vi "OpenProject.vi"() -> ()   [LabVIEW 2020]
uses:
  <vilib>/Wiresmith Technology/G CLI/CLI Class/CLI.lvclass
panel:
  out "String":string
  out "Error out":errorcluster
  in  "Project_Path":path=path "C:/Workspace/Git/PVS_2.0/SourceCode/PVS_BE/Projects/PVS_BE.lvproj"
  in  "Error_In":errorcluster
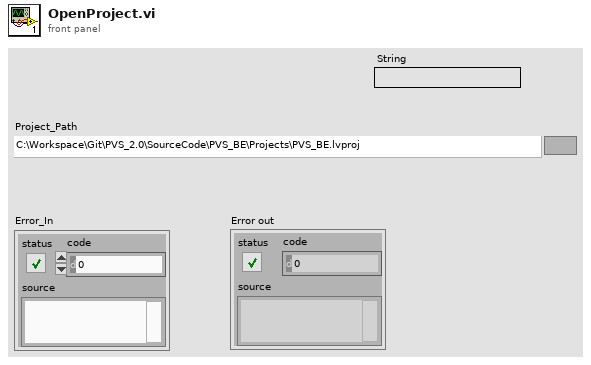
[diagram p1: front panel]
types:
  T1 = enum32{"Invalid", "Standard", "Closed", "Hidden", "Minimized", "Maximized"}
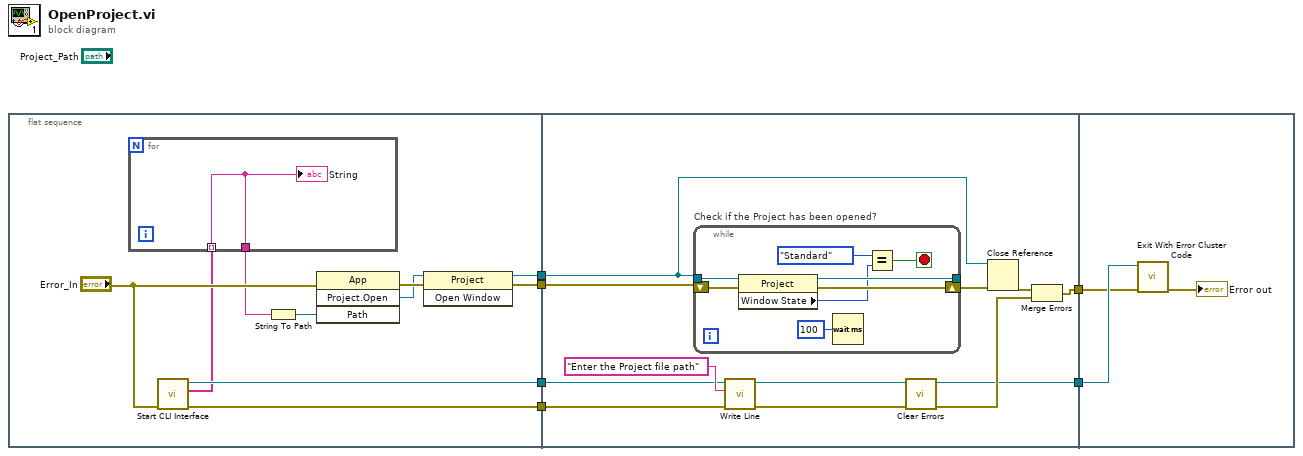
[diagram p0: block diagram]
diagram:
  n1 = flat-sequence {
    tunnel: [w14] -> w4
    tunnel: [w13] -> w3
    tunnel: [w12] -> w2
    tunnel: [w11] -> w1
    tunnel: [w18] -> w6
    tunnel: [w24] -> w5
    tunnel: w4 -> [w26]
    tunnel: w3 -> [w25]
    tunnel: w2 -> [w22]
    tunnel: w1 -> [w20]
    tunnel: w6 -> [w39]
    tunnel: w5 -> [w38]
    frame #0 {
      n2 = call <vilib>:"Start CLI Interface.vi"("error in (no error)"="Error_In") -> ("error out"=w12:errorcluster, "Custom Parameters"=w9:string[], "CLI out"=w11:refnum<class "CLI.lvclass">)  [unwired: 7 in, 1 out]
      n3 = for {
        tunnel: w9 -> [w17] mode=indexing
        tunnel: [w17] -> w8
        "String" <- w17
      }
      n4 = String To Path(string=w8) -> (path=w7:path)
      n5 = invoke class="App" method="Project.Open"(error in="Error_In", "Path"=w7) -> (error out=w16:errorcluster, "Project:Open"=w15:refnum<vi>)  [unwired: 2 in, 2 out]
      n6 = invoke class="Project" method="Open Window"(reference=w15, error in=w16) -> (reference out=w13:refnum<vi>, error out=w14:errorcluster)  [unwired: 1 in, 1 out]
    }
    frame #1 {
      n7 = while "Check if the Project has been opened?" {
        tunnel: [w34] -> _
        shift-right: [w35] -> w27
        shift-left: w26 -> [w30]
        tunnel: w25 -> [w29]
        stop <- w31 stop-if-true
        n8 = property class="Project"(reference=w29, error in=w30) -> (reference out=w34:refnum<vi>, error out=w35:errorcluster, "Window State"=w33:T1)
        n9 = Wait (ms)(milliseconds to wait=u32 100) -> ()  [unwired: 1 out]
        n10 = Equal?(x=T1."Standard" ("Window State 2"), y=w33) -> (x = y?=w31:bool)
      }
      n11 = call <vilib>:"Write Line.vi"("error in (no error)"=w22, "Text to Write"="Enter the Project file path", "CLI in"=w20) -> ("error out"=w23:errorcluster, "CLI out"=w18:refnum<class "CLI.lvclass">)  [unwired: 7 in]
      n12 = call <vilib>:"Clear Errors.vi"("error in (no error)"=w23) -> ("error out"=w19:errorcluster)  [unwired: 5 in, 1 out]
      n13 = Close Reference(reference=w25, error in (no error)=w27) -> (error out=w28:errorcluster)
      n14 = Merge Errors(w28, w19) -> (w24:errorcluster)
    }
    frame #2 {
      n15 = call <vilib>:"Exit With Error Cluster Code.vi"("error in (no error)"=w38, "CLI in"=w39) -> ("error out"=→"Error out":errorcluster)  [unwired: 9 in]
    }
  }
